vi "lv_icon.vi"(8 "error in (no error)":errorcluster, 9 "BW icon in":T1, 10 "Color icon in":T1, 11 "_lv_icon_class in":refnum<class "lv_icon_class.lvclass">) -> (0 "error out":errorcluster, 1 "Color icon out":T1, 2 "BW icon out":T1, 3 "_lv_icon_class out":refnum<class "lv_icon_class.lvclass">, 4 "Error code out":i32)   [LabVIEW 2021, in "lv_icon_class.lvclass"]
uses:
  <vilib>/LabVIEW Icon API/lv_icon/lv_icon_class/lv_icon_class.lvclass
  <vilib>/LabVIEW Icon API/lv_icon/lv_icon_class/lv_icon_class.lvclass/lv_icon_class.ctl
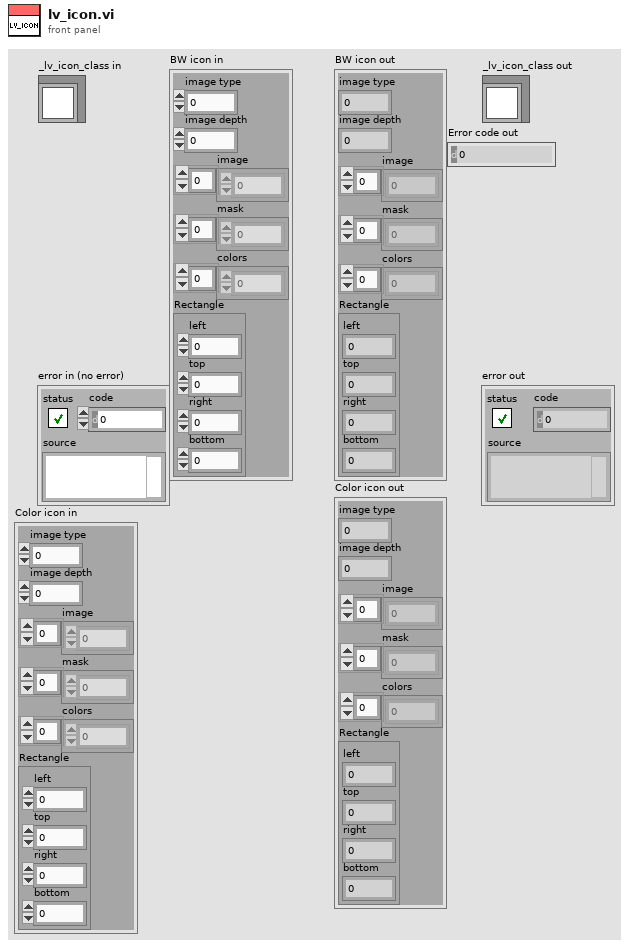
[diagram p1: front panel]
types:
  T1 = cluster{"image type":i32, "image depth":i32, "image":u8[], "mask":u8[], "colors":u32[], "Rectangle":cluster{"left":i16, "top":i16, "right":i16, "bottom":i16}}
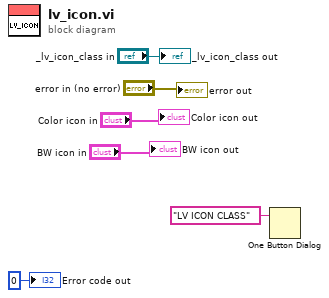
[diagram p0: block diagram]
diagram:
  n1 = One Button Dialog(message="LV ICON CLASS") -> ()  [unwired: 1 in, 1 out]
  "error out" <- "error in (no error)"
  "_lv_icon_class out" <- "_lv_icon_class in"
  "BW icon out" <- "BW icon in"
  "Color icon out" <- "Color icon in"
  "Error code out" <- 0 ("Error code out")
